vi "Is Open.vi"(8 "error in (no error)":errorcluster, 11 "TCPResource in":refnum<class "TCPResource.lvclass">) -> (0 "error out":errorcluster, 2 "Is Open":bool, 3 "TCPResource out":refnum<class "TCPResource.lvclass">)   [LabVIEW 2020, in "PicoG-Core.lvlib" / "TCPResource.lvclass"]
uses:
  TCPResource.lvclass
  TCPResource.lvclass/TCPResource.ctl
  <vilib>/IlluminatedG/lv-stream-tcp/TCP Client/TCP Client.lvclass
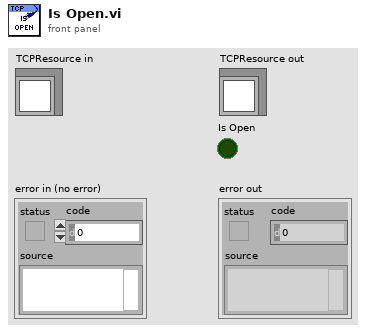
[diagram p1: front panel]
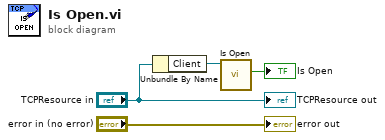
[diagram p0: block diagram]
diagram:
  n1 = Unbundle By Name("TCPResource in") -> ("Client"=w2:refnum<class "TCP Client.lvclass">)
  n2 = call-dynamic "Is Open.vi"("TCP Client in"=w2) -> ("Is Open"=→"Is Open":bool)  [unwired: 8 in, 2 out]
  "error out" <- "error in (no error)"
  "TCPResource out" <- "TCPResource in"
